vi "Initiate.vi"(8 "error in (no error)":errorcluster, 11 "VISA resource name":refnum<visa-resource-name>) -> (0 "error out":errorcluster, 3 "VISA resource name out":refnum<visa-resource-name>)   [LabVIEW 2013]
doc: "This VI initiates output changes that you previously specified.\n\nIf the power supply is not currently waiting for a trigger, the power supply waits for the trigger you specify with the hpe364xa Configure Trigger Source VI after you call this VI. After the power supply detects the trigger, it updates its voltage level and current limit to the values you specify with the hpe364xa Configure Triggered Voltage Lev and hpe364xa Configure Triggered Current Lim VIs.\n\n\nIf the power supply is already waiting for a trigger, this VI does nothing."
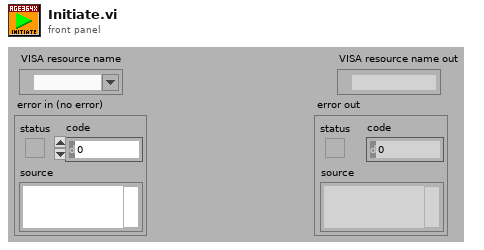
[diagram p1: front panel]
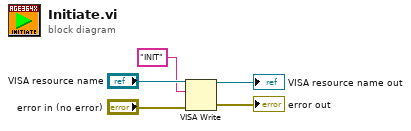
[diagram p0: block diagram]
diagram:
  n1 = VISA Write(VISA resource name="VISA resource name", write buffer="INIT", error in (no error)="error in (no error)") -> (VISA resource name out=→"VISA resource name out":refnum<visa-resource-name>, error out=→"error out":errorcluster)  [unwired: 1 out]
